vi "FileRefFGV.vi"(10 "Action":T1(ring), 11 "File in":path) -> (2 "Changed?":bool, 3 "File out":path)   [LabVIEW 2012, in "StimulCtrls.lvlib"]
uses:
  StimulCtrls.lvlib
panel:
  # "This VI is to save File I/O, and to check if SEQ content is changed."
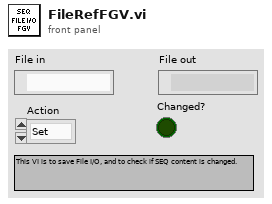
[diagram p1: front panel]
types:
  T1 = enum16{"Set", "Get", "Initial", "Change", "Saved"}
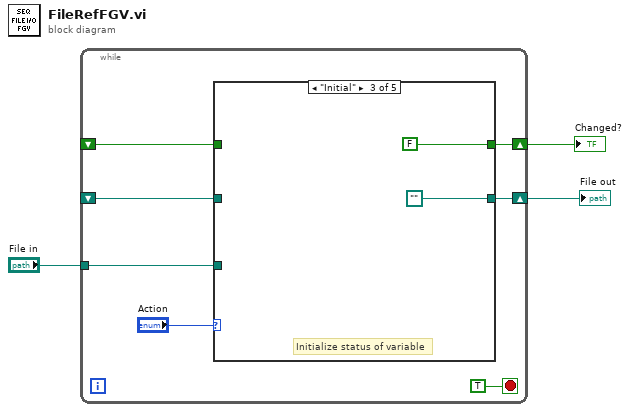
[diagram p0: block diagram]
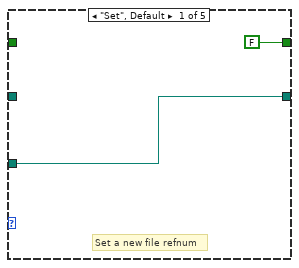
[diagram p2: hidden frame]
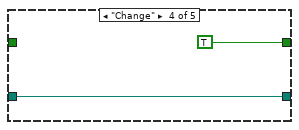
[diagram p4: hidden frame]
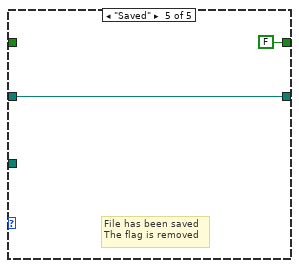
[diagram p5: hidden frame]
diagram:
  n1 = while {
    tunnel: "File in" -> [w6]
    shift-right: [w9] -> w1
    shift-left: _ -> [w8]
    shift-right: [w5] -> w3
    shift-left: _ -> [w4]
    stop <- TRUE stop-if-true
    n2 = case shown="\"Initial\"" "Action" {
      tunnel: [w12 w14 path "" w18 w20] -> w9
      tunnel: w6 -> [w12 _ _ _ _]
      tunnel: w8 -> [_ w14 _ w18 w20]
      tunnel: [FALSE w13 FALSE TRUE FALSE] -> w5
      tunnel: w4 -> [_ w13 _ _ _]
      frame "Set", Default {
        # "Set a new file refnum"
      }
      frame "Get" {
      }
      frame "Initial" {
        # "Initialize status of variable"
      }
      frame "Change" {
      }
      frame "Saved" {
        # "File has been saved\nThe flag is removed"
      }
    }
  }
  "Changed?" <- w3
  "File out" <- w1
